vi "Init Events.vi"(8 "error in (no error)":errorcluster, 11 "TSEngine in":refnum<class "Engine.lvclass">) -> (0 "error out":errorcluster, 3 "TSEngine out":refnum<class "Engine.lvclass">, 4 "Event Reg":refnum<event-registration>, 6 "Events":T1)   [LabVIEW 2020, in "TSS.lvlib" / "Engine.lvclass"]
uses:
  Engine.lvclass
  Events.ctl
  Create VC Event Data.ctl
  Variable Container Type.ctl
  VariableContainer/Typedefs/Session Handle.ctl
  VariableContainer/VariableContainer.lvclass
  Create Report Event Data.ctl
  Execution/Typedefs/Session Handle.ctl
  Execution/Execution.lvclass
  Report/Typedefs/Session Handle.ctl
  Report/Report.lvclass
  Engine.lvclass/Engine.ctl
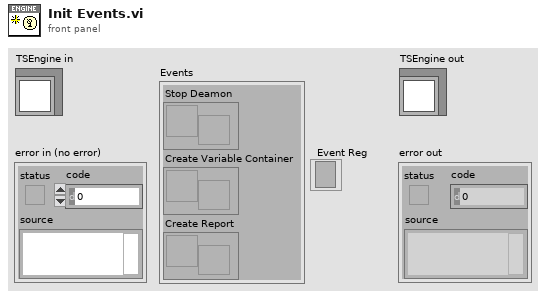
[diagram p1: front panel]
types:
  T1 = typedef "TSS.lvlib/Engine.lvclass/Events.ctl" = cluster{"Stop Deamon":refnum<user-event>, "Create Variable Container":refnum<user-event>, "Create Report":refnum<user-event>}
  T2 = typedef "TSS.lvlib/Engine.lvclass/Create Report Event Data.ctl" = cluster{"Execution":T3, "Report Notifier":refnum<notifier>}
  T3 = typedef "TSS.lvlib/Execution.lvclass/Session Handle.ctl" = refnum<data-value>
  T4 = typedef "TSS.lvlib/Engine.lvclass/Create VC Event Data.ctl" = cluster{"Type":T5, "Notifier":refnum<notifier>}
  T5 = typedef "TSS.lvlib/Engine.lvclass/Variable Container Type.ctl" = enum16{"StationGlobals", "TemporaryGlobals", "NewPropertyObject"}
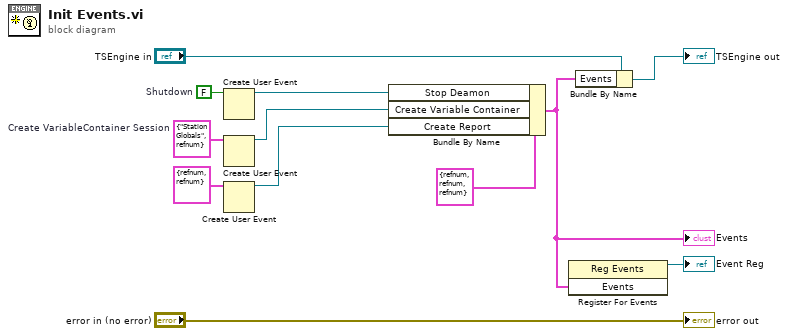
[diagram p0: block diagram]
diagram:
  w10 = T4 {"Type"=enum."StationGlobals", "Notifier"=refnum}  # Create VariableContainer Session
  w11 = FALSE  # Shutdown
  n1 = Create User Event(user event datatype=w11) -> (user event=w7:refnum<user-event>)  [unwired: 1 in, 1 out]
  n2 = Create User Event(user event datatype=w10) -> (user event=w6:refnum<user-event>)  [unwired: 1 in, 1 out]
  n3 = Create User Event(user event datatype=T2 {"Execution"=refnum, "Report Notifier"=refnum} ("Create Report Event Data")) -> (user event=w1:refnum<user-event>)  [unwired: 1 in, 1 out]
  n4 = Bundle By Name(cluster=T1 {"Stop Deamon"=refnum, "Create Variable Container"=refnum, "Create Report"=refnum} ("Events"), "Stop Deamon"=w7, "Create Variable Container"=w6, "Create Report"=w1) -> (w4:T1)
  "Events" <- w4
  n5 = register-events(w4) -> (reference out=→"Event Reg":refnum<event-registration>)  [unwired: 2 in, 1 out]
  n6 = Bundle By Name(cluster="TSEngine in", "Events"=w4) -> (→"TSEngine out":refnum<class "Engine.lvclass">)
  "error out" <- "error in (no error)"
